vi "MDPtr DAQ Example(obsolete).vi"() -> ()   [LabVIEW 2017]
uses:
  MDPtr TypeDef/MDPtr SupportedDataTypeDef.ctl
  MDPtr TypeDef/MDPtr.ctl
  _PolymorphicVIs/MDPtr Unpack Waveform.vi
  _PolymorphicVIs/MDPtr Pack Waveform.vi
  MDPtr.lvlib
  <vilib>/measure/NI_MABase.lvlib
  _MDPtrMgr/MDPtrMgr.lvclass
panel:
  out "# elements in queue":i32
  out "Value out":i64
  out "File Logging?":bool
  out "MDPtr Total Count":i64
  in  "file path":path=path "D:/MDPtr.tdms"
  out "Square":waveform(dbl)(graph)
  out "Sine":waveform(dbl)(graph)
  in  "stop":bool
  out "Copy Count":i32
  out "Data Type":T1
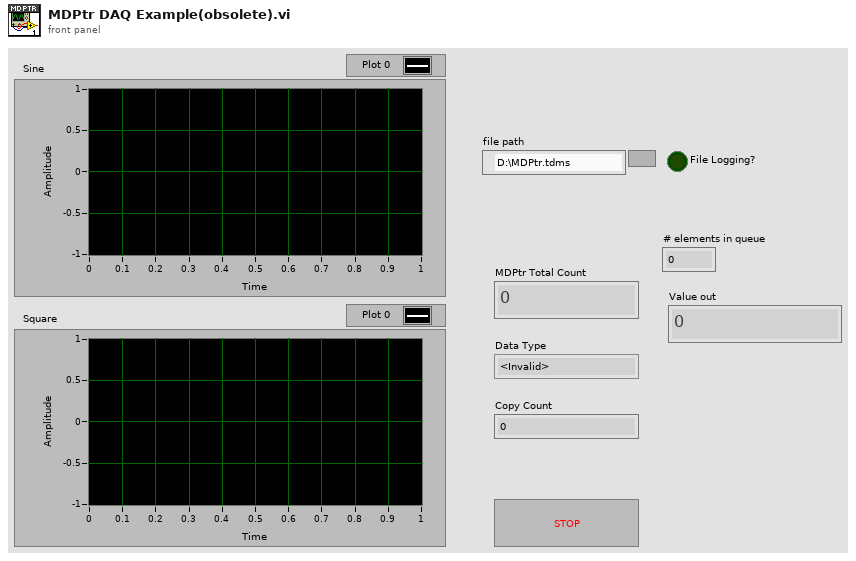
[diagram p1: front panel]
types:
  T1 = typedef "MDPtr.lvlib/MDPtr SupportedDataTypeDef.ctl" = enum16{"<Invalid>", "<User 0>", "<User 1>", "<User 2>", "<User 3>", "<User 4>", "Memory", "Waveform", "Waveform Arr", "Double Arr", "String Arr"}
  T2 = enum16{"open", "open or create", "create or replace", "create", "open (read-only)"}
  T3 = typedef "MDPtr.lvlib/MDPtr.ctl" = refnum<k1>
  T4 = typedef "MDPtr.lvlib/Def-MDPtrQueue.ctl" = refnum<queue>
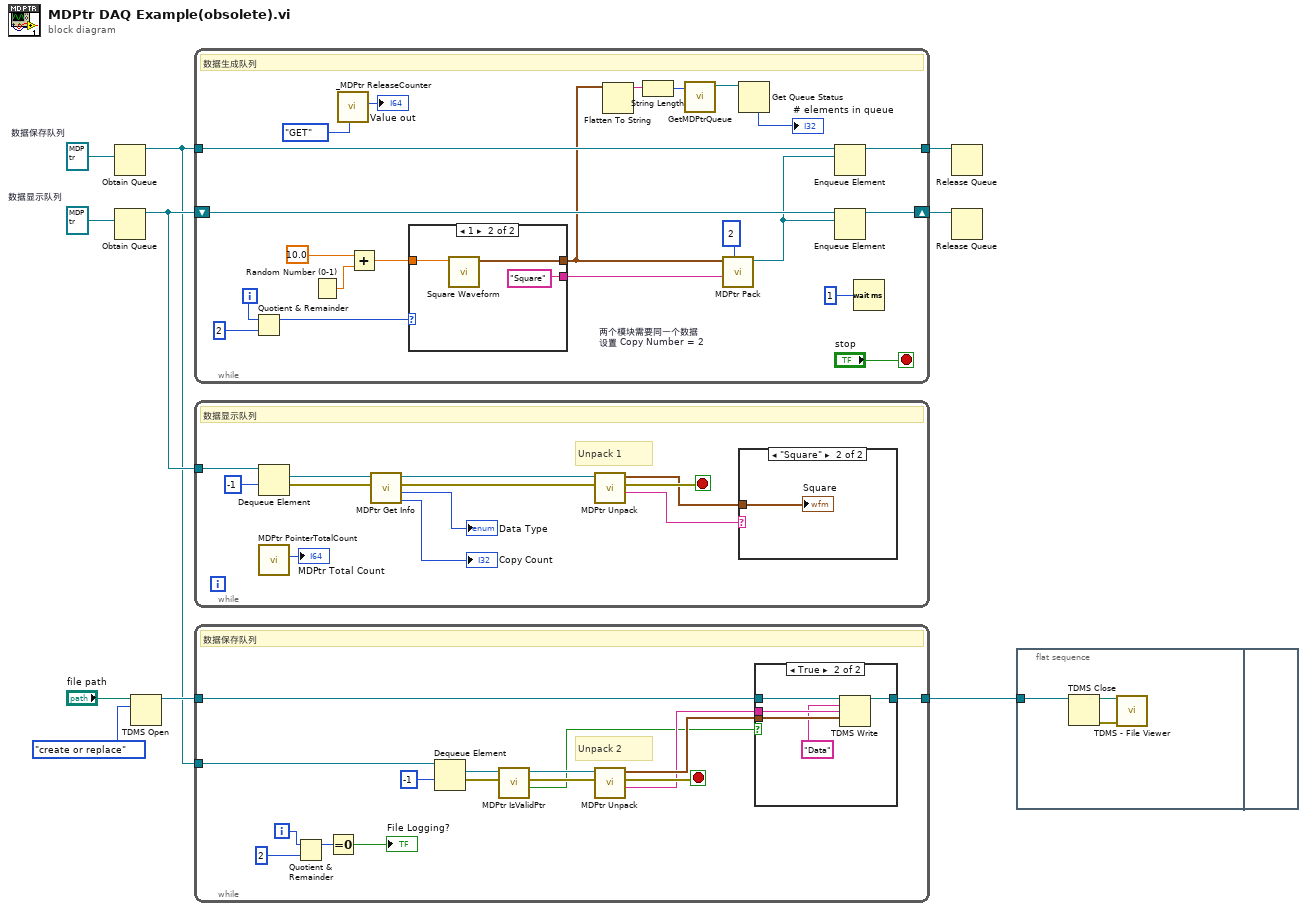
[diagram p0: block diagram]
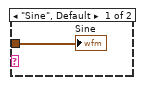
[diagram p3: hidden frame]
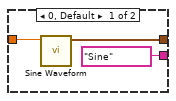
[diagram p4: hidden frame]
diagram:
  n1 = Obtain Queue "数据保存队列"(element data type=T3 refnum ("MDPtr")) -> (queue out=w3:refnum<queue>)  [unwired: 4 in, 2 out]
  n2 = Obtain Queue "数据显示队列"(element data type=T3 refnum ("MDPtr")) -> (queue out=w7:refnum<queue>)  [unwired: 4 in, 2 out]
  n3 = TDMS Open(10:T2."create or replace" ("operation (0:open)"), 11:"file path") -> (3:w5:refnum<k34>)  [unwired: 5 in, 1 out]
  n4 = while {
    shift-right: [w31] -> w1
    shift-left: w7 -> [w32]
    tunnel: w3 -> [w20]
    tunnel: [w19] -> w2
    i -> [w29]
    stop <- "stop" stop-if-true
    w21 = 2  # 两个模块需要同一个数据 设置 Copy Number = 2
    # "数据生成队列"
    n5 = Quotient & Remainder(x=w29, y=2) -> (x-y*floor(x/y)=w27:i32)  [unwired: 1 out]
    n6 = Random Number (0-1)() -> (number: 0 to 1=w23:dbl)
    n7 = call "_MDPtr ReleaseCounter.vi"("Oper(Get)"=enum16{"GET", "Increament", "decreament"}."GET") -> ("Value out"=→"Value out":i64)  [unwired: 9 in, 1 out]
    n8 = Add(x=10.0 ("frequency"), y=w23) -> (x+y=w22:dbl)
    n9 = case shown="1" w27 {
      tunnel: [w35 w38] -> w12
      tunnel: ["Sine" ("String Attribute") "Square" ("String Attribute")] -> w26
      tunnel: w22 -> [w33 w36]
      frame 0, Default {
        n10 = call <vilib>:"Sine Waveform.vi"("frequency"=w33) -> ("signal out"=w35:waveform(dbl))  [unwired: 9 in, 1 out]
      }
      frame 1 {
        n11 = call <vilib>:"Square Waveform.vi"("frequency"=w36) -> ("signal out"=w38:waveform(dbl))  [unwired: 9 in, 1 out]
      }
    }
    n12 = Flatten To String(anything=w12) -> (data string=w11:string)  [unwired: 3 in, 2 out]
    n13 = String Length(string=w11) -> (length=w13:i32)
    n14 = call "GetMDPtrQueue.vi"("MemoryLength"=w13) -> ("MDPtrQueue"=w14:T4)  [unwired: 9 in, 1 out]
    n15 = call-poly "MDPtr Pack.vi"("Copies Count(1)"=w21, "String Attribute"=w26, "waveform"=w12) -> ("HexStrPtr"=w18:T3)  [unwired: 7 in, 1 out]
    n16 = Get Queue Status(queue=w14) -> (# elements in queue=→"# elements in queue":i32)  [unwired: 2 in, 7 out]
    n17 = Enqueue Element(queue=w20, element=w18) -> (queue out=w19:refnum<queue>)  [unwired: 2 in, 2 out]
    n18 = Enqueue Element(queue=w32, element=w18) -> (queue out=w31:refnum<queue>)  [unwired: 2 in, 2 out]
    n19 = Wait (ms)(milliseconds to wait=u32 1) -> ()  [unwired: 1 out]
  }
  n20 = while {
    tunnel: w7 -> [w50]
    stop <- w48 stop-if-true
    # "Unpack 1"
    # "数据显示队列"
    n21 = Dequeue Element(queue=w50, timeout in ms (-1)=-1) -> (element=w40:T3, error out=w46:errorcluster)  [unwired: 1 in, 2 out]
    n22 = call "MDPtr PointerTotalCount.vi"() -> ("MDPtr Total Count"=→"MDPtr Total Count":i64)  [unwired: 10 in, 1 out]
    n23 = call "MDPtr Get Info.vi"("error in (no error)"=w46, "HexStrPtr"=w40) -> ("Copy Count"=→"Copy Count":i32, "Data Type"=→"Data Type":T1, "error out"=w45:errorcluster, "HexStrPtr (dup)"=w43:T3)  [unwired: 5 in, 1 out]
    n24 = call-poly "MDPtr Unpack.vi"("error in (no error)"=w45, "HexStrPtr"=w43) -> ("String Attribute"=w42:string, "error out"=w48:errorcluster, "waveform"=w41:waveform(dbl))  [unwired: 7 in]
    n25 = case shown="\"Square\"" w42 {
      tunnel: w41 -> [w51 w52]
      frame "Sine", Default {
        "Sine" <- w51
      }
      frame "Square" {
        "Square" <- w52
      }
    }
  }
  n26 = while {
    tunnel: w3 -> [w68]
    tunnel: [w63] -> w6
    tunnel: w5 -> [w64]
    i -> [w55]
    stop <- w66 stop-if-true
    # "Unpack 2"
    # "数据保存队列"
    n27 = Quotient & Remainder(x=w55, y=2) -> (x-y*floor(x/y)=w54:i32)  [unwired: 1 out]
    n28 = Equal To 0?(x=w54) -> (x = 0?=→"File Logging?":bool)
    n29 = Dequeue Element(queue=w68, timeout in ms (-1)=-1) -> (element=w65:T3, error out=w58:errorcluster)  [unwired: 1 in, 2 out]
    n30 = call "MDPtr IsValidPtr.vi"("error in (no error)"=w58, "HexStrPtr"=w65) -> ("Valid MDPtr?"=w57:bool, "error out"=w59:errorcluster, "HexStrPtr (dup)"=w60:T3)  [unwired: 6 in]
    n31 = call-poly "MDPtr Unpack.vi"("error in (no error)"=w59, "HexStrPtr"=w60) -> ("String Attribute"=w61:string, "error out"=w66:errorcluster, "waveform"=w62:waveform(dbl))  [unwired: 7 in]
    n32 = case shown="True" w57 {
      tunnel: w64 -> [w69 w74]
      tunnel: [w69 w73] -> w63
      tunnel: w62 -> [_ w72]
      tunnel: w61 -> [_ w71]
      frame False {
      }
      frame True {
        n33 = TDMS Write(0:w74, 5:"Data" ("group name in (Untitled)"), 7:w71, 9:w72) -> (4:w73:refnum<k34>)  [unwired: 2 in, 3 out]
      }
    }
  }
  n34 = Release Queue(queue=w2) -> ()  [unwired: 2 in, 3 out]
  n35 = Release Queue(queue=w1) -> ()  [unwired: 2 in, 3 out]
  n36 = flat-sequence {
    tunnel: w6 -> [w77]
    frame #0 {
      n37 = TDMS Close(11:w77) -> (0:w76:errorcluster, 3:w75:path)  [unwired: 1 in]
      n38 = call <vilib>:"TDMS - File Viewer.vi"("error in (no error)"=w76, "file path"=w75) -> ()  [unwired: 4 in, 2 out]
    }
    frame #1 {
    }
  }
